vi "Build_Argument_String.vi"(1 "Flow Array":dbl[](array[numeric]), 2 "Argument List":string[](array[string]), 3 "Command":string) -> (0 "Argument String":string)   [LabVIEW 2011]
doc: "This VI takes a Command (string), an Argument List (array of strings) and a Flow Array (array of doubles) and outputs a single string that is useful for writing to a log or saving to a file. This VI uses the appropriate syntax to allow the parsing VIs to read the data. The syntax is as follows:\n\nCommand:Boolean_Argument,Text_Argument(\"some text\"),Flow_Argument(\"12.3\")\n\nNote that this VI does not store a time value. In growth sequence files, the time value is stored as plaintext after the the last argument, separated by a single space character. This functionality is implemented in a higher-level VI."
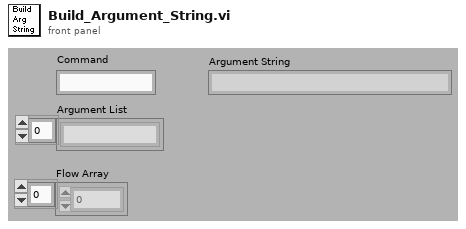
[diagram p1: front panel]
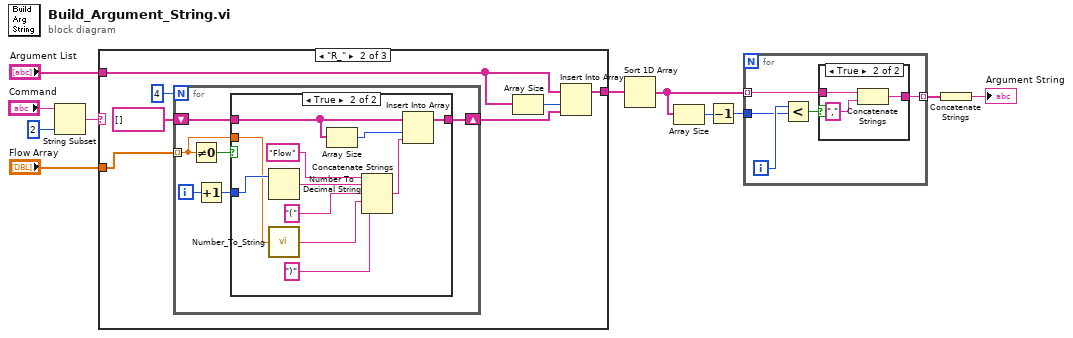
[diagram p0: block diagram]
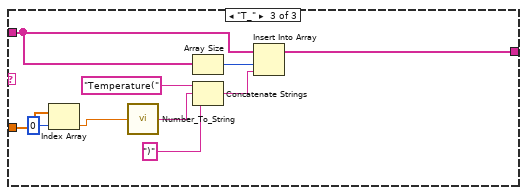
[diagram p4: hidden frame]
diagram:
  n1 = String Subset(string="Command", length (rest)=2 ("length (rest)")) -> (substring=w6:string)  [unwired: 1 out]
  n2 = case shown="\"R_\"" w6 {
    tunnel: "Flow Array" -> [_ w18 w46]
    tunnel: "Argument List" -> [w12 w15 w42]
    tunnel: [w12 w13 w40] -> w2
    frame Default {
    }
    frame "R_" {
      n3 = for {
        N: 4 -> [_]
        tunnel: w18 -> [w24] mode=indexing
        shift-right: [w23] -> w16
        shift-left: string[] [] -> [w22]
        i -> [w21]
        n4 = Not Equal To 0?(x=w24) -> (x != 0?=w25:bool)
        n5 = Increment(x=w21) -> (x+1=w20:i32)
        n6 = case shown="True" w25 {
          tunnel: w24 -> [_ w27]
          tunnel: [w26 w32] -> w23
          tunnel: w22 -> [w26 w30]
          tunnel: w20 -> [_ w29]
          frame False {
          }
          frame True {
            n7 = Number To Decimal String(number=w29) -> (decimal integer string=w36:string)  [unwired: 1 out]
            n8 = call "Number_To_String.vi"("Number"=w27) -> ("String"=w28:string)
            n9 = Array Size(array=w30) -> (size(s)=w31:i32)
            n10 = Concatenate Strings("Flow", w36, "(" ("string"), w28, ")" ("string")) -> (w33:string)
            n11 = Insert Into Array(array=w30, index=w31, new element=w33) -> (w32:string[])
          }
        }
      }
      n12 = Array Size(array=w15) -> (size(s)=w14:i32)
      n13 = Insert Into Array(array=w15, index=w14, new element=w16) -> (w13:string[])
    }
    frame "T_" {
      n14 = Index Array(array=w46, index=0) -> (element=w38:dbl)
      n15 = call "Number_To_String.vi"("Number"=w38) -> ("String"=w39:string)
      n16 = Array Size(array=w42) -> (size(s)=w43:i32)
      n17 = Concatenate Strings("Temperature(" ("string"), w39, ")" ("string")) -> (w41:string)
      n18 = Insert Into Array(array=w42, index=w43, new element=w41) -> (w40:string[])
    }
  }
  n19 = Sort 1D Array(array=w2) -> (sorted array=w1:string[])
  n20 = Array Size(array=w1) -> (size(s)=w11:i32)
  n21 = Decrement(x=w11) -> (x-1=w10:i32)
  n22 = for {
    tunnel: w1 -> [w52] mode=indexing
    tunnel: [w51] -> w3 mode=indexing
    tunnel: w10 -> [w48]
    i -> [w49]
    n23 = Less?(x=w49, y=w48) -> (x < y?=w50:bool)
    n24 = case shown="True" w50 {
      tunnel: w52 -> [w53 w56]
      tunnel: [w53 w54] -> w51
      frame False {
      }
      frame True {
        n25 = Concatenate Strings(w56, "," ("string")) -> (w54:string)
      }
    }
  }
  n26 = Concatenate Strings(w3) -> (→"Argument String":string)
